vi "Master test.vi"() -> ()   [LabVIEW 2015]
uses:
  Source files/Typedefs/Dynamic report parameters.ctl
  <vilib>/vision/Image Controls.llb/IMAQ Image.ctl
panel:
  in  "Batch details":string[][](array[string])=[["A", "1.234", "2.345", "3.456", "4.567", "5.678"], ["B", "2.345", "4.556", "5.678", "6.678", "9.987"], ["C", "2.234", "4.456", "1.123", "2.234", "3.345"], ["D", "6.678", "1.123", "2.234", "4.456", "3.345"], ["E", "3.345", "4.456", "5.567", "6.678", "7.789"]]
  in  "Part details":string[][](array[string])=[["A", "1.234", "2.345", "3.456", "4.567", "5.678", "mm", "PASS"], ["B", "2.345", "4.556", "5.678", "6.678", "9.987", "mm", "PASS"], ["C", "2.234", "4.456", "1.123", "2.234", "3.345", "mm", "FAIL"], ["D", "6.678", "1.123", "2.234", "4.456", "3.345", "mm", "PASS"], ["E", "3.345", "4.456", "5.567", "6.678", "7.789", "mm", "PASS"]]
  in  "Print?":bool
  in  "Part image filepath":path=path "E:/Temporary Code Modification/TEX based report generation/Project/Image files/Test images/Part1.png"
  in  "Yield chart filepath":path=path "E:/Temporary Code Modification/TEX based report generation/Project/Image files/YieldChart.png"
  in  "ZenReport configuration filepath":path=path "E:/Temporary Code Modification/Test outputs/Test results/ZenReport configuration v1.0.2.json"
  in  "Report type":string(combo)="Part"
  out "Detailed error out":string
  out "error out":errorcluster
  in  "error in (no error)":errorcluster
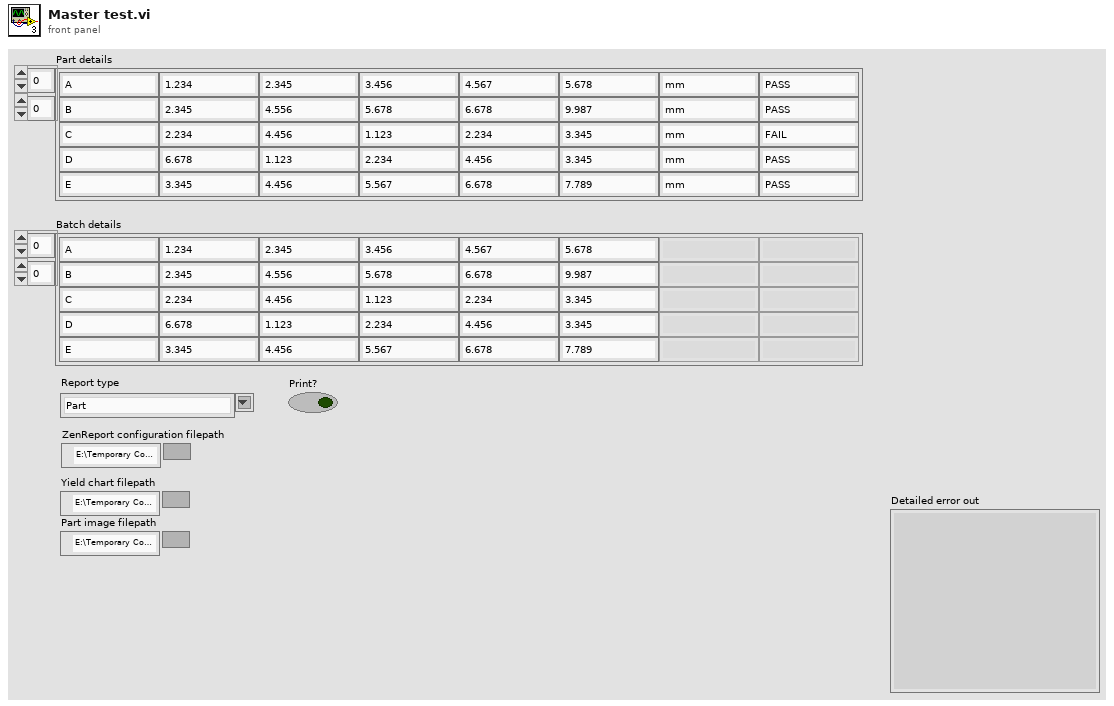
[diagram p1: front panel]
types:
  T1 = cluster{"Table ID":string, "Table data":string[][]}
  T2 = typedef "IMAQ Image.ctl" = refnum<image>
  T3 = typedef "Image Type" = u32
  T4 = typedef "Dynamic report parameters.ctl" = cluster{"Part name":string, "Batch ID (optional)":string, "Report type":string, "Operator name":string, "Job number":string, "Measurement Data and Time":string, "Report name prefix":string, "Inspection status":bool, "Bookmarks":cluster{"Bookmark key":string, "Bookmark value":string}[], "Image parameters":cluster{"Image ID":string, "Image":T2}[], "Table parameters":cluster{"Table ID":string, "Table data":string[][]}}
  T5 = typedef "ZenReport private.ctl" = cluster{"JSON Variant":variant, "Output PDF filepath":string, "Printer name":string, "Run until completion (PDF generate)":bool, "Run minimized (PDF generate)":bool, "Run until completion (print)":bool, "Run minimized (print)":bool}
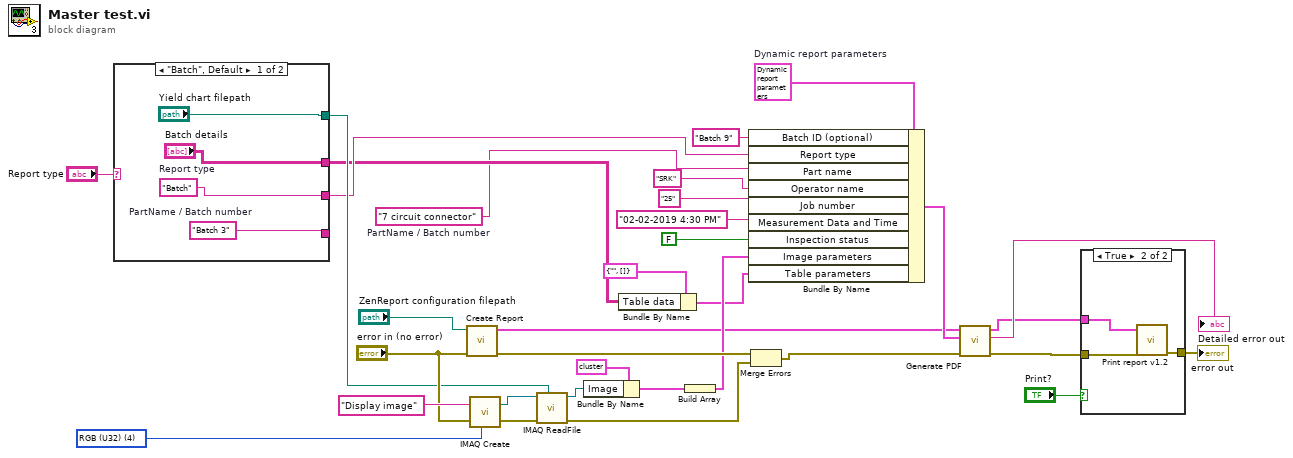
[diagram p0: block diagram]
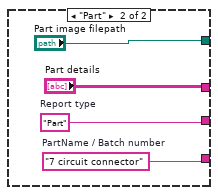
[diagram p3: hidden frame]
diagram:
  w1 = "7 circuit connector"  # PartName / Batch number
  w25 = T3 4 items=["Grayscale (U8)", "Grayscale (I16)", "Grayscale (SGL)", "Complex (CSG)", "RGB (U32)", "HSL (U32)", "RGB (U64)", "Grayscale (U16)"] ("Image Type")
  w32 = T4 {"Part name"="", "Batch ID (optional)"="", "Report type"="", "Operator name"="", "Job number"="", "Measurement Data and Time"="", "Report name prefix"="", "Inspection status"=FALSE, "Bookmarks"=[], "Image parameters"=[], "Table parameters"={"Table ID"="", "Table data"=[]}}  # Dynamic report parameters
  n1 = case shown="\"Batch\", Default" "Report type" {
    tunnel: ["Yield chart filepath" "Part image filepath"] -> w12
    tunnel: ["Batch details" "Part details"] -> w4
    tunnel: [w36 w40] -> w11
    tunnel: [w35 w39] -> _
    frame "Batch", Default {
      w35 = "Batch 3"  # PartName / Batch number
      w36 = "Batch"  # Report type
    }
    frame "Part" {
      w39 = "7 circuit connector"  # PartName / Batch number
      w40 = "Part"  # Report type
    }
  }
  n2 = call "Create Report.vi"("error in (no error)"="error in (no error)", "ZenReport configuration filepath"="ZenReport configuration filepath") -> ("error out"=w20:errorcluster, "ZenReport public data"=w9:T5)  [unwired: 8 in]
  n3 = call "IMAQ Create"("Image Name"="Display image", "Image Type"=w25, "error in (no error)"="error in (no error)") -> ("New Image"=w23:T2, "error out"=w24:errorcluster)  [unwired: 2 in]
  n4 = call "IMAQ ReadFile"("File Path"=w12, "error in (no error)"=w24, "Image"=w23) -> ("error out"=w18:errorcluster, "Image Out"=w21:T2)  [unwired: 4 in, 3 out]
  n5 = Bundle By Name(cluster=cluster{"Image ID":string, "Image":T2} {"Image ID"="", "Image"=refnum} ("Bookmark details"), "Image"=w21) -> (w17:cluster{"Image ID":string, "Image":T2})
  n6 = Bundle By Name(cluster=T1 {"Table ID"="", "Table data"=[]} ("Table parameters"), "Table data"=w4) -> (w2:T1)
  n7 = Build Array(w17) -> (w16:cluster{"Image ID":string, "Image":T2}[])
  n8 = Bundle By Name(cluster=w32, "Batch ID (optional)"="Batch 9", "Report type"=w11, "Part name"=w1, "Operator name"="SRK", "Job number"="25", "Measurement Data and Time"="02-02-2019 4:30 PM", "Inspection status"=FALSE, "Image parameters"=w16, "Table parameters"=w2) -> (w15:T4)
  n9 = Merge Errors(w20, w18) -> (w19:errorcluster)
  n10 = call "Generate PDF.vi"("error in"=w19, "Dynamic report parameters"=w15, "ZenReport private"=w9) -> ("error out"=w6:errorcluster, "Detailed error out"=→"Detailed error out":string, "ZenReport private data"=w7:T5)  [unwired: 6 in]
  n11 = case shown="True" "Print?" {
    tunnel: [w42 w45] -> w8
    tunnel: w7 -> [_ w44]
    tunnel: w6 -> [w42 w43]
    frame False {
    }
    frame True {
      n12 = call "Print report v1.2.vi"("error in"=w43, "ZenReport public data"=w44) -> ("error out"=w45:errorcluster)  [unwired: 9 in]
    }
  }
  "error out" <- w8
